vi "Year2019 Q1.vi"() -> ()   [LabVIEW 2018]
panel:
  out "sum of n elements":dbl
  out "nth element":dbl
  in  "n":dbl
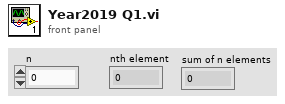
[diagram p1: front panel]
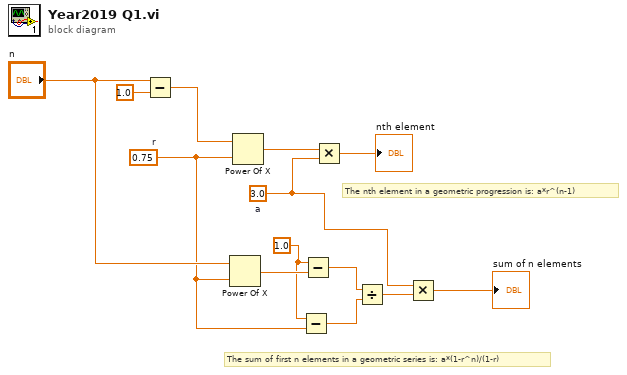
[diagram p0: block diagram]
diagram:
  w7 = 1.0 ("x")
  w1 = 3.0  # a
  w6 = 0.75  # r
  # "The sum of first n elements in a geometric series is: a*(1-r^n)/(1-r)"
  # "The nth element in a geometric progression is: a*r^(n-1)"
  n1 = Subtract(x="n", y=1.0) -> (x-y=w12:dbl)
  n2 = Power Of X(1:w6, 2:"n") -> (0:w8:dbl)
  n3 = Power Of X(1:w6, 2:w12) -> (0:w11:dbl)
  n4 = Subtract(x=w7, y=w6) -> (x-y=w4:dbl)
  n5 = Subtract(x=w7, y=w8) -> (x-y=w5:dbl)
  n6 = Multiply(x=w11, y=w1) -> (x*y=→"nth element":dbl)
  n7 = Divide(x=w5, y=w4) -> (x/y=w3:dbl)
  n8 = Multiply(x=w1, y=w3) -> (x*y=→"sum of n elements":dbl)
